vi "Apply.vi"(8 "error in":errorcluster, 11 "DAQmx Thermocouple Continuous Read Strategy in":refnum<class "DAQmx Thermocouple Continuous Read Strategy.lvclass">) -> (0 "error out":errorcluster, 3 "DAQmx Thermocouple Continuous Read Strategy out":refnum<class "DAQmx Thermocouple Continuous Read Strategy.lvclass">)   [LabVIEW 2024, in "DAQmx Thermocouple Continuous Read Strategy.lvclass"]
uses:
  DAQmx Thermocouple Continuous Read Strategy.lvclass
  DAQmx Thermocouple Continuous Read Strategy.lvclass/DAQmx Thermocouple Continuous Read Strategy.ctl
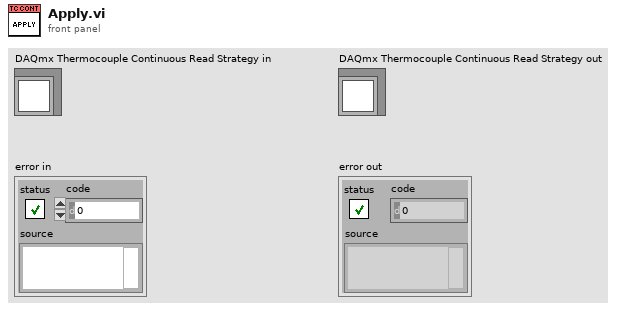
[diagram p1: front panel]
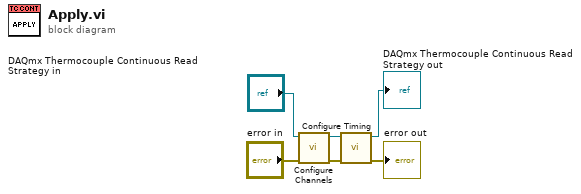
[diagram p0: block diagram]
diagram:
  n1 = call-dynamic "Configure Channels.vi"("error in"="error in", "DAQmx Thermocouple Continuous Read Strategy in"="DAQmx Thermocouple Continuous Read Strategy in") -> ("error out"=w4:errorcluster, "DAQmx Thermocouple Continuous Read Strategy out"=w3:refnum<class "DAQmx Thermocouple Continuous Read Strategy.lvclass">)  [unwired: 8 in]
  n2 = call-dynamic "Configure Timing.vi"("error in"=w4, "DAQmx Base Configure Strategy in"=w3) -> ("error out"=→"error out":errorcluster, "DAQmx Base Configure Strategy out"=→"DAQmx Thermocouple Continuous Read Strategy out":refnum<class "DAQmx Thermocouple Continuous Read Strategy.lvclass">)  [unwired: 8 in]
